vi "Beta 1.2.vi"() -> ()   [LabVIEW 2011]
panel:
  out "XY Graph":cluster{dbl[], dbl[]}(graph)
  out "Original Image":T1(plugin-control)
  out "Path to Image":path
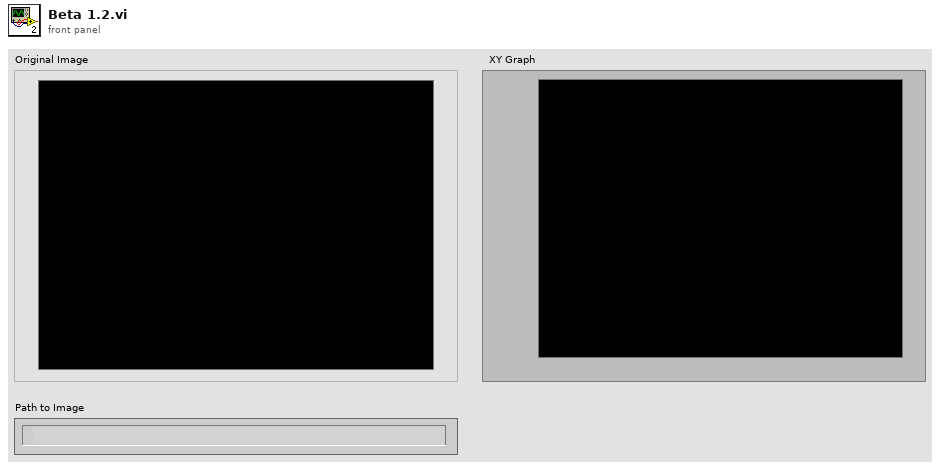
[diagram p1: front panel]
types:
  T1 = typedef "IMAQ Image.ctl" = refnum<image>
  T2 = typedef "Image Type" = u32
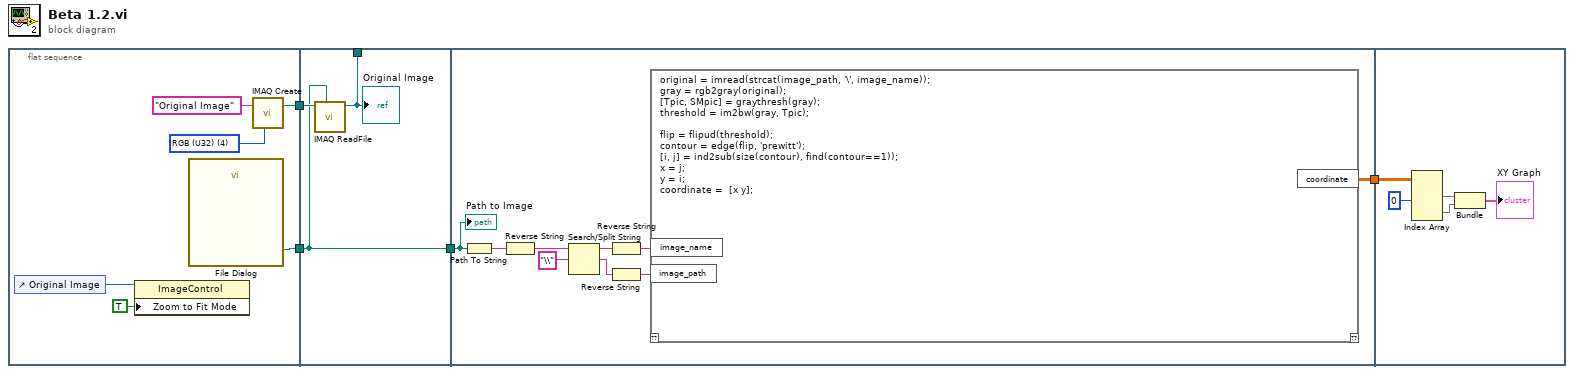
[diagram p0: block diagram]
diagram:
  n1 = flat-sequence {
    tunnel: [w6] -> w4
    tunnel: [w5] -> w3
    tunnel: w4 -> [w13]
    tunnel: w3 -> [w12]
    tunnel: [w12] -> w2
    tunnel: [w11] -> _
    tunnel: w2 -> [w15]
    tunnel: [w14] -> w1
    tunnel: w1 -> [w27]
    frame #0 {
      w8 = T2 4 items=["Grayscale (U8)", "Grayscale (I16)", "Grayscale (SGL)", "Complex (CSG)", "RGB (U32)", "HSL (U32)", "RGB (U64)", "Grayscale (U16)"] ("Image Type")
      n2 = control-ref of="Original Image"() -> (w9:refnum<vi>)
      n3 = property class="ImageControl"(reference=w9, "Zoom to Fit Mode"=TRUE) -> ()  [unwired: 1 in, 2 out]
      n4 = call "File Dialog"() -> ("selected path"=w5:path)  [unwired: 12 in, 3 out]
      n5 = call "IMAQ Create"("Image Name"="Original Image", "Image Type"=w8) -> ("New Image"=w6:T1)  [unwired: 3 in, 1 out]
    }
    frame #1 {
      n6 = call "IMAQ ReadFile"("File Path"=w12, "Image"=w13) -> ("Image Out"=w11:T1)  [unwired: 5 in, 4 out]
      "Original Image" <- w11
    }
    frame #2 {
      n7 = Path To String(path=w15) -> (string=w22:string)
      n8 = Reverse String(1:w22) -> (0:w21:string)
      n9 = Search/Split String(string=w21, search string/char (-)="\\") -> (substring before match=w19:string, match + rest of string=w18:string)  [unwired: 1 in, 1 out]
      n10 = Reverse String(1:w19) -> (0:w17:string)
      n11 = Reverse String(1:w18) -> (0:w16:string)
      n12 = script code="original = imread(strcat(image_path, '\\', image_name));\ngray = rgb2gray(original);\n[Tpic, SMpic] = graythresh(gray);\nthreshold = im2bw(gray, Tpic);\n\nflip = flipud(threshold);\ncontour = edge(flip, 'prewitt');\n[i, j] = ind2sub(size(contour), find(contour==1));\nx = j;\ny = i;\ncoordinate =  [x y];"("image_name"=w17, "image_path"=w16) -> ("coordinate"=w14:dbl[][])  [unwired: 1 in, 1 out]
      "Path to Image" <- w15
    }
    frame #3 {
      n13 = Index Array(array=w27, index (col) #1=0 ("disabled index (col)")) -> (element #1=w25:dbl[], element #2=w24:dbl[])  [unwired: 3 in]
      n14 = Bundle(w25, w24) -> (→"XY Graph":cluster{dbl[], dbl[]})  [unwired: 1 in]
    }
  }
